vi "Hierarchical VArray to MultiD Array.vi"(8 "error in (no error)":errorcluster, 9 "Element Type":variant, 10 "Hierarchical Array":variant[](array[variant]), 11 "Deserializer in":refnum<class "JSON Deserializer.lvclass">) -> (0 "error out":errorcluster, 2 "MultiD Array":variant, 3 "Deserializer out":refnum<class "JSON Deserializer.lvclass">)   [LabVIEW 2020, in "JKI JSON Serialization.lvlib" / "JSON Deserializer.lvclass"]
uses:
  JSON Deserializer.lvclass
  JSON Deserializer.lvclass/JSON Deserializer.ctl
  <vilib>/Utility/Data Type/NI_Data Type.lvlib
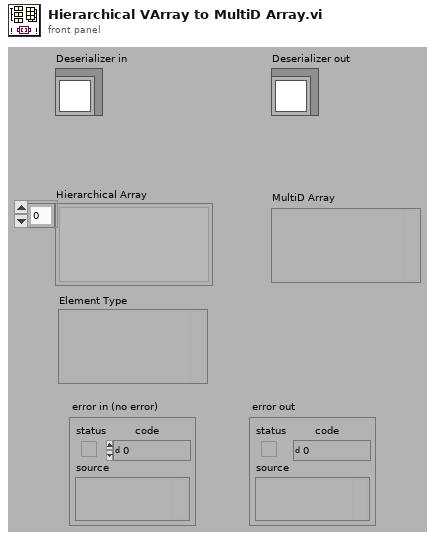
[diagram p1: front panel]
types:
  T1 = typedef "NI_Data Type.lvlib/Data Type.ctl" = enum8{"Invalid Type", "Void", "I8", "I16", "I32", "I64", "U8", "U16", "U32", "U64", "Single Float", "Double Float", "Extended Float", "Single Complex", "Double Complex", "Extended Complex", "Enum U8", "Enum U16", "Enum U32", "Enum U64", "Single Float With Unit", "Double Float With Unit", "Extended Float With Unit", "Single Complex with Unit", "Double Complex with Unit", "Extended Complex with Unit", "Boolean", "String", "Path", "Picture", "Tag", "Array", "Cluster", "Variant", "LV Variant", "Waveform", "Timestamp", "Digital Waveform", "Digital Data", "ExpressData", "Refnum", "External Data", "VI", "Poly VI", "LabVIEW Class Instance", "Fixed Point", "Set Collection", "Map Collection"}
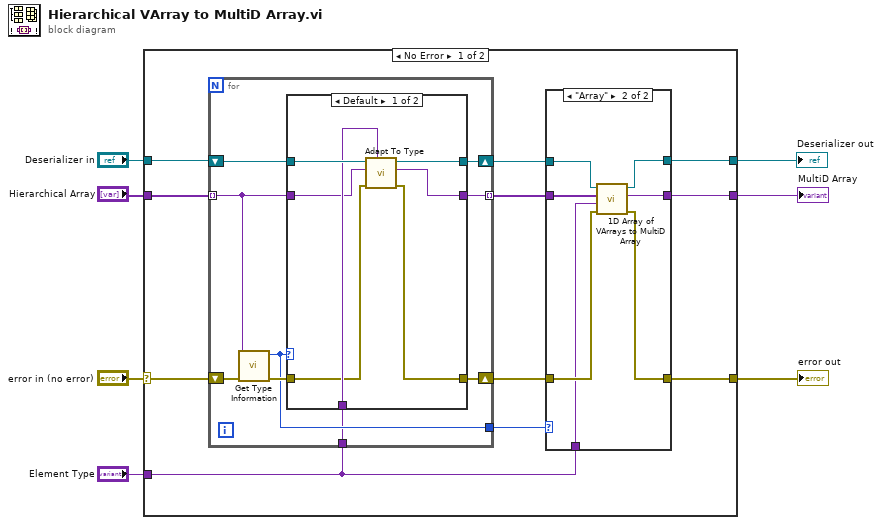
[diagram p0: block diagram]
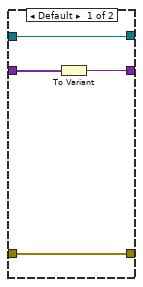
[diagram p2: hidden frame]
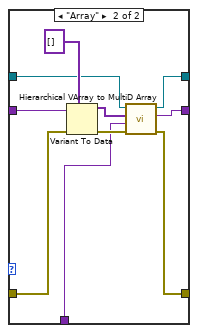
[diagram p3: hidden frame]
diagram:
  n1 = case shown="No Error" "error in (no error)" {
    selector: "error in (no error)" -> [w17 w57]
    tunnel: [w14 w57] -> w7
    tunnel: [w13 _] -> w4
    tunnel: "Hierarchical Array" -> [w18 _]
    tunnel: "Element Type" -> [w11 _]
    tunnel: "Deserializer in" -> [w10 w56]
    tunnel: [w8 w56] -> w1
    frame No Error {
      n2 = for {
        tunnel: w18 -> [w35] mode=indexing
        shift-right: [w37] -> w15
        shift-left: w17 -> [w38]
        tunnel: [w34] -> w16 mode=indexing
        tunnel: [w33] -> w12
        tunnel: w11 -> [w32]
        shift-right: [w30] -> w9
        shift-left: w10 -> [w31]
        n3 = call <vilib>:"Get Type Information.vi"("error in (no error)"=w38, "variant"=w35) -> ("error out"=w36:errorcluster, "type"=w33:T1)  [unwired: 5 in, 3 out]
        n4 = case shown="Default" w33 {
          tunnel: [w39 w50] -> w37
          tunnel: w36 -> [w40 w49]
          tunnel: w35 -> [w42 w55]
          tunnel: [w41 w51] -> w34
          tunnel: w32 -> [w43 w46]
          tunnel: w31 -> [w45 w48]
          tunnel: [w44 w47] -> w30
          frame Default {
            n5 = call-dynamic "Adapt To Type.vi"("Type and Defaults"=w43, "error in (no error)"=w40, "Variant in"=w42, "Deserializer in"=w45) -> ("error out"=w39:errorcluster, "Variant out"=w41:variant, "Deserializer out"=w44:refnum<class "JSON Deserializer.lvclass">)  [unwired: 5 in]
          }
          frame "Array" {
            n6 = Variant To Data(error in=w49, type=variant[] [], Variant=w55) -> (data=w53:variant[], error out=w52:errorcluster)
            n7 = call "Hierarchical VArray to MultiD Array.vi"("error in (no error)"=w52, "Element Type"=w46, "Hierarchical Array"=w53, "Deserializer in"=w48) -> ("error out"=w50:errorcluster, "MultiD Array"=w51:variant, "Deserializer out"=w47:refnum<class "JSON Deserializer.lvclass">)  [unwired: 5 in]
          }
        }
      }
      n8 = case shown="\"Array\"" w12 {
        tunnel: w16 -> [w21 w29]
        tunnel: w15 -> [w20 w28]
        tunnel: [w20 w27] -> w14
        tunnel: [w22 w26] -> w13
        tunnel: w11 -> [_ w25]
        tunnel: w9 -> [w19 w24]
        tunnel: [w19 w23] -> w8
        frame Default {
          n9 = To Variant(anything=w21) -> (Variant=w22:variant)
        }
        frame "Array" {
          n10 = call "1D Array of VArrays to MultiD Array.vi"("error in (no error)"=w28, "Element Type"=w25, "Array of VArrays"=w29, "Deserializer in"=w24) -> ("error out"=w27:errorcluster, "MultiD Array"=w26:variant, "Deserializer out"=w23:refnum<class "JSON Deserializer.lvclass">)  [unwired: 5 in]
        }
      }
    }
    frame Error {
    }
  }
  "error out" <- w7
  "MultiD Array" <- w4
  "Deserializer out" <- w1
